vi "BaseConverter.vi"(6 "Action":bool=TRUE, 8 "Base":dbl=16.0, 11 "Input":dbl) -> (3 "Output":i16=16384)   [LabVIEW 2016]
doc: "Input: the number to be converted \nBase: maximum amplitude the number can be\nAction: FALSE to convert from FXP to Natural and TRUE to convert from Natural to FXP"
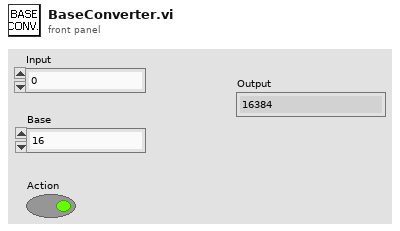
[diagram p1: front panel]
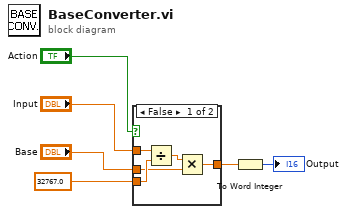
[diagram p0: block diagram]
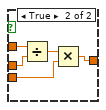
[diagram p2: hidden frame]
diagram:
  n1 = case shown="False" "Action" {
    tunnel: "Input" -> [w11 w16]
    tunnel: "Base" -> [w7 w14]
    tunnel: [w8 w13] -> w2
    tunnel: 32767.0 ("y") -> [w10 w12]
    frame False {
      n2 = Divide(x=w11, y=w10) -> (x/y=w9:dbl)
      n3 = Multiply(x=w9, y=w7) -> (x*y=w8:dbl)
    }
    frame True {
      n4 = Divide(x=w16, y=w14) -> (x/y=w15:dbl)
      n5 = Multiply(x=w15, y=w12) -> (x*y=w13:dbl)
    }
  }
  n6 = To Word Integer(number=w2) -> (16bit integer=→"Output":i16)
